vi "Create.vi"(8 "error in (no error)":errorcluster, 9 "Name Map In":map{string, i32}(c390), 10 "Values":refnum<class "Type.lvclass">[](array[class])) -> (0 "error out":errorcluster, 1 "Name Map":map{string, i32}(c390), 3 "Result Row out":refnum<class "Result Row.lvclass">)   [LabVIEW 2022 SP3, in "Conditum.lvlib" / "Result Row.lvclass"]
uses:
  Result Row.lvclass
  Columns/Type/Type.lvclass
  Columns/Type/Type.lvclass/Type.ctl
  Result Row.lvclass/Result Row.ctl
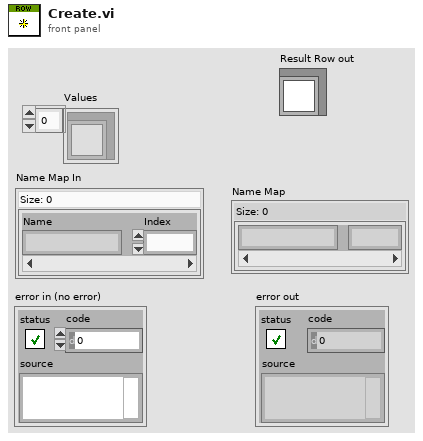
[diagram p1: front panel]
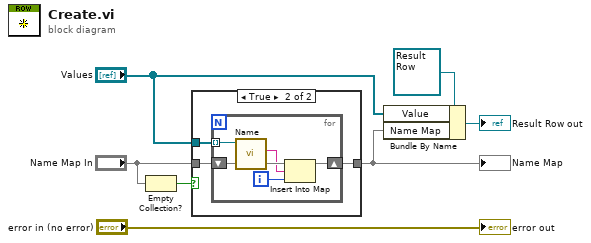
[diagram p0: block diagram]
diagram:
  n1 = Empty Collection?(1:"Name Map In") -> (0:w5:bool)
  n2 = case shown="True" w5 {
    tunnel: "Values" -> [_ w10]
    tunnel: "Name Map In" -> [w8 w11]
    tunnel: [w8 w9] -> w2
    frame False {
    }
    frame True {
      n3 = for {
        shift-right: [w12] -> w9
        shift-left: w11 -> [w16]
        tunnel: w10 -> [w15] mode=indexing
        i -> [w13]
        n4 = call "Name.vi"("Type in"=w15) -> ("Table Name"=w14:string)  [unwired: 10 in]
        n5 = Insert Into Map(map in=w16, key=w14, value=w13) -> (map out=w12:map{string, i32})  [unwired: 2 out]
      }
    }
  }
  "Name Map" <- w2
  n6 = Bundle By Name(cluster=refnum<class "Result Row.lvclass"> refnum ("Result Row out"), "Value"="Values", "Name Map"=w2) -> (→"Result Row out":refnum<class "Result Row.lvclass">)
  "error out" <- "error in (no error)"
